vi "24HP_Clone.vi"(0 "Single 24HP":T1) -> (2 "DAQ Error":errorcluster, 3 "All samples out":sgl[][](array[numeric]), 4 "Ch No":i16[](array[numeric]), 5 "Index":i32[](array[numeric]), 6 "Sampling Rate Hz":dbl)   [LabVIEW 2020]
doc: "Use this plug-in with the Nathan 7609 data acquisition system"
uses:
  Device ID port info.ctl
  ctls/24HP_Cmd (USB).ctl
  Globals/Meas_global.vi
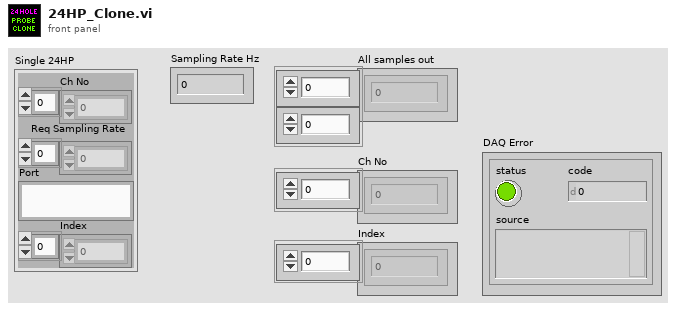
[diagram p1: front panel]
types:
  T1 = typedef "Device ID port info.ctl" = cluster{"Ch No":i16[], "Req Sampling Rate":dbl[], "Port":string, "Index":i32[]}
  T2 = typedef "24HP_Cmd (USB).ctl" = string
  T3 = typedef "24HP_Data cluster.ctl" = cluster{"Time stamp":timestamp, "Pressures (Pa)":sgl[], "T_external (°C)":sgl, "T_board (°C)":sgl, "P_atm (mbar)":sgl, "Rel. hum. (%)":sgl, "a_xyz (g)":sgl[], "w_xyz (dps)":sgl[], "Status bytes":u8[]}
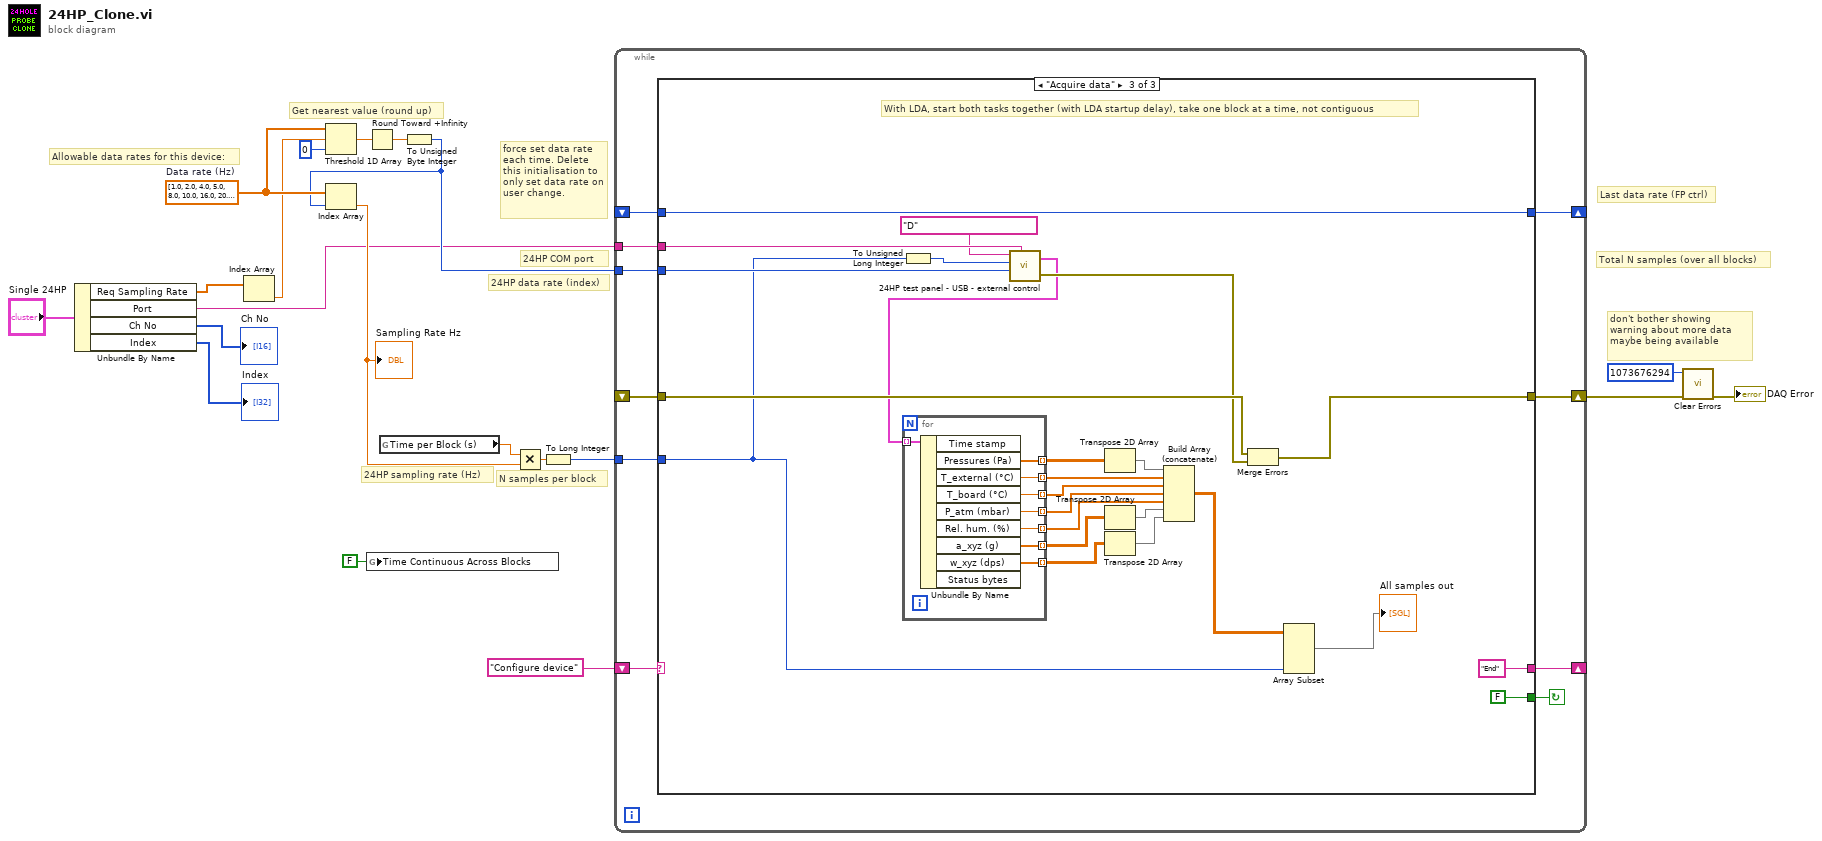
[diagram p0: block diagram]
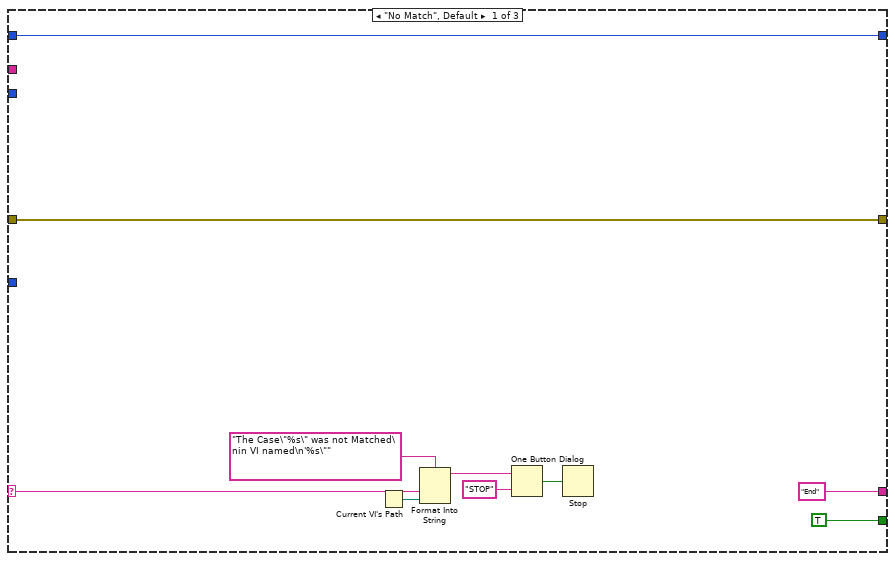
[diagram p2: hidden frame]
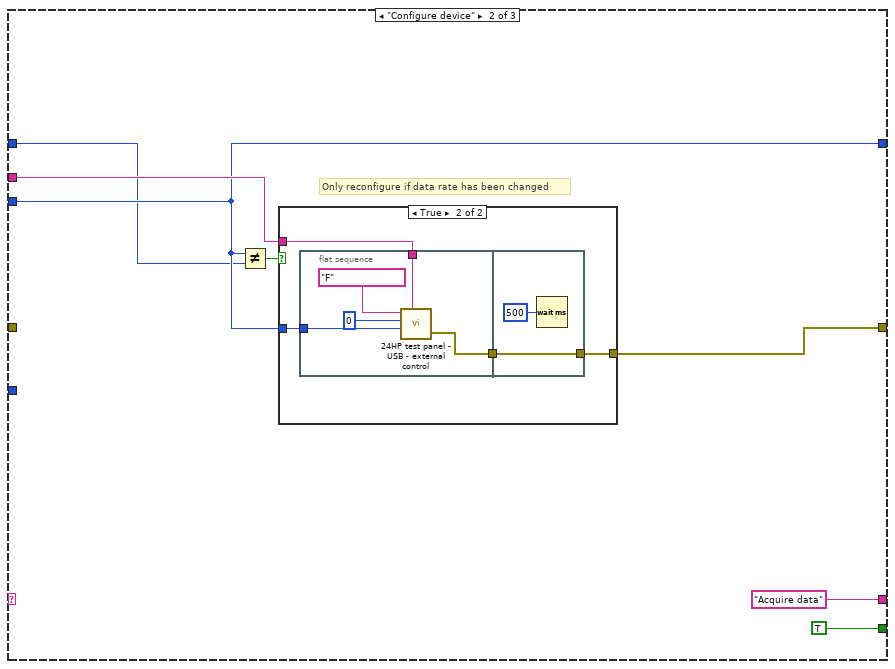
[diagram p3: hidden frame]
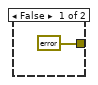
[diagram p4: hidden frame]
diagram:
  w14 = dbl[] [1.0, 2.0, 4.0, 5.0, 8.0, 10.0, 16.0, 20.0, 25.0, 32.0, 40.0, 50.0, 64.0, 80.0, 100.0, 125.0, 160.0, 200.0, 250.0, 320.0, 400.0, 500.0, 625.0, 800.0, 1000.0]  # Data rate (Hz)
  # "N samples per block"
  # "24HP sampling rate (Hz)"
  # "24HP COM port"
  # "24HP data rate (index)"
  # "Allowable data rates for this device:"
  # "Get nearest value (round up)"
  # "force set data rate each time. Delete this initialisation to only set data rate on user change."
  # "Last data rate (FP ctrl)"
  # "Total N samples (over all blocks)"
  # "don't bother showing warning about more data maybe being available"
  n1 = Unbundle By Name("Single 24HP") -> ("Req Sampling Rate"=w5:dbl[], "Port"=w6:string, "Ch No"=→"Ch No":i16[], "Index"=→"Index":i32[])
  n2 = Index Array(array=w5) -> (element=w4:dbl)  [unwired: 1 in]
  n3 = Threshold 1D Array(1:0 ("start index (0)"), 2:w4, 3:w14) -> (0:w15:dbl)
  n4 = Round Toward +Infinity(x=w15) -> (ceil(x): smallest int >= x=w13:dbl)
  n5 = global write "Meas_global.vi" "Time Continuous Across Blocks"(FALSE ("Time Continuous Across Blocks")) -> ()
  n6 = global read "Meas_global.vi" "Time per Block (s)"() -> (w12:dbl)
  n7 = To Unsigned Byte Integer(number=w13) -> (unsigned 8bit integer=w8:u8)
  n8 = Index Array(array=w14, index=w8) -> (element=w9:dbl)
  "Sampling Rate Hz" <- w9
  n9 = Multiply(x=w12, y=w9) -> (x*y=w11:dbl)
  n10 = To Long Integer(number=w11) -> (32bit integer=w10:i32)
  n11 = while {
    shift-left: "Configure device" -> [w30]
    shift-right: [w25] -> _
    tunnel: w10 -> [w29]
    shift-right: [w26] -> w17
    shift-left: _ -> [w27]
    tunnel: w6 -> [w24]
    tunnel: w8 -> [w23]
    shift-right: [w22] -> _
    shift-left: _ -> [w21]
    stop <- w28 continue-if-true
    n12 = case shown="\"Acquire data\"" w30 {
      selector: w30 -> [w33 _ _]
      tunnel: ["End" "Acquire data" ("f") "End"] -> w25
      tunnel: w29 -> [_ _ w60]
      tunnel: [TRUE TRUE FALSE] -> w28
      tunnel: w27 -> [w32 _ w81]
      tunnel: [w32 w46 w80] -> w26
      tunnel: w24 -> [_ w44 w79]
      tunnel: w23 -> [_ w43 w78]
      tunnel: [w31 w43 w77] -> w22
      tunnel: w21 -> [w31 w42 w77]
      frame "No Match", Default {
        n13 = Current VI's Path() -> (path=w36:path)
        n14 = Format Into String(format string="The Case\"%s\" was not Matched\nin VI named\n'%s\"" ("Format String"), w33, w36) -> (resulting string=w39:string)  [unwired: 2 in, 1 out]
        n15 = One Button Dialog(message=w39, button name ("OK")="STOP") -> (true=w37:bool)
        n16 = Stop(stop? (T)=w37) -> ()
      }
      frame "Configure device" {
        # "Only reconfigure if data rate has been changed"
        n17 = Not Equal?(x=w43, y=w42) -> (x != y?=w41:bool)
        n18 = case shown="True" w41 {
          tunnel: [errorcluster {"status"=FALSE, "code"=0, "source"=""} ("error IO") w51] -> w46
          tunnel: w44 -> [_ w50]
          tunnel: w43 -> [_ w52]
          frame False {
          }
          frame True {
            n19 = flat-sequence {
              tunnel: w52 -> [w55]
              tunnel: w50 -> [w53]
              tunnel: [w54] -> w49
              tunnel: [w59] -> w51
              tunnel: w49 -> [w59]
              frame #0 {
                n20 = call "24HP test panel - USB - external control.vi"("COM port"=w53, "Data rate (Hz)"=w55, "N samples"=u32 0, "Command"=T2 "F") -> ("Error"=w54:errorcluster)  [unwired: 2 in, 1 out]
              }
              frame #1 {
                n21 = Wait (ms)(milliseconds to wait=u32 500) -> ()  [unwired: 1 out]
              }
            }
          }
        }
      }
      frame "Acquire data" {
        # "With LDA, start both tasks together (with LDA startup delay), take one block at a time, not contiguous"
        n22 = To Unsigned Long Integer(number=w60) -> (unsigned 32bit integer=w75:u32)
        n23 = call "24HP test panel - USB - external control.vi"("COM port"=w79, "Data rate (Hz)"=w78, "N samples"=w75, "Command"=T2 "D") -> ("Error"=w76:errorcluster, "Data out"=w74:T3[])  [unwired: 2 in]
        n24 = for {
          tunnel: w74 -> [w91] mode=indexing
          tunnel: [w90] -> w68 mode=indexing
          tunnel: [w89] -> w73 mode=indexing
          tunnel: [w88] -> w72 mode=indexing
          tunnel: [w87] -> w71 mode=indexing
          tunnel: [w86] -> w70 mode=indexing
          tunnel: [w85] -> w64 mode=indexing
          tunnel: [w84] -> w66 mode=indexing
          n25 = Unbundle By Name(w91) -> ("Pressures (Pa)"=w90:sgl[], "T_external (°C)"=w89:sgl, "T_board (°C)"=w88:sgl, "P_atm (mbar)"=w87:sgl, "Rel. hum. (%)"=w86:sgl, "a_xyz (g)"=w85:sgl[], "w_xyz (dps)"=w84:sgl[])  [unwired: 2 out]
        }
        n26 = Transpose 2D Array(2D array=w68) -> (transposed array=w67:sgl[][])
        n27 = Transpose 2D Array(2D array=w64) -> (transposed array=w63:sgl[][])
        n28 = Transpose 2D Array(2D array=w66) -> (transposed array=w65:sgl[][])
        n29 = Build Array (concatenate)(w67, w73, w72, w71, w70, w63, w65) -> (w62:sgl[][])
        n30 = Merge Errors(w81, w76) -> (w80:errorcluster)
        n31 = Array Subset(array=w62, length (col)=w60) -> (→"All samples out":sgl[][])  [unwired: 3 in]
      }
    }
  }
  n32 = call <vilib>:"Clear Errors.vi"("error in (no error)"=w17, "specific error code to clear (0: all)"=1073676294) -> ("error out"=→"DAQ Error":errorcluster)  [unwired: 4 in, 1 out]
